vi "Atto DRY Interface is Persistent Mode Set.vi"(8 "error in (no error)":errorcluster, 11 "PersistentMode":i32) -> (0 "error out":errorcluster, 2 "function return":i32, 3 "PersistentMode out":i32)   [LabVIEW 2016, in "attoDRYLib.lvlib"]
doc: "int32_t __cdecl AttoDRY_Interface_isPersistentModeSet(\n int *PersistentMode);"
uses:
  <userlib>/attoDRYLib/attoDRYLib.lvlib
  <userlib>/attoDRYLib/attoDRYLib.dll
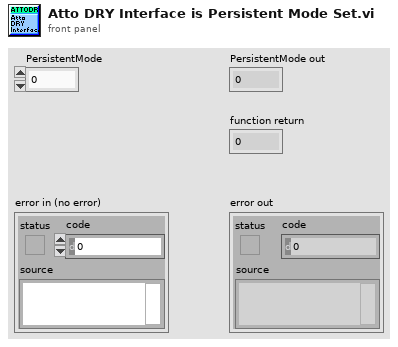
[diagram p1: front panel]
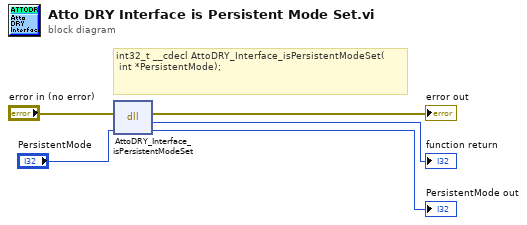
[diagram p0: block diagram]
diagram:
  # "int32_t __cdecl AttoDRY_Interface_isPersistentModeSet(\n\tint *PersistentMode);"
  n1 = dll-call lib="C:/Program Files (x86)/National Instruments/LabVIEW 2016/user.lib/attoDRYLib/attoDRYLib.*" fn="AttoDRY_Interface_isPersistentModeSet"(error in="error in (no error)", "PersistentMode"="PersistentMode") -> (error out=→"error out":errorcluster, →"function return":i32, "PersistentMode"=→"PersistentMode out":i32)  [unwired: 2 in, 1 out]
